vi "Configure AIN U6.vi"(4 "Binary":bool, 5 "Ranges":string[](array[string]), 6 "SettlingFactor":i32, 7 "Positive Channels":i32[](array[numeric]), 8 "error in":errorcluster, 10 "Resolution":i32, 11 "Handle In":i32) -> (0 "error out":errorcluster, 3 "Handle Out":i32)   [LabVIEW 2020]
panel:
  # "Pass an array of channels and range constants for\nthose channels."
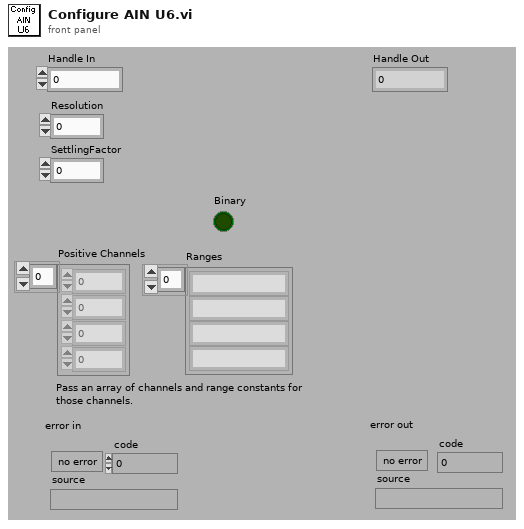
[diagram p1: front panel]
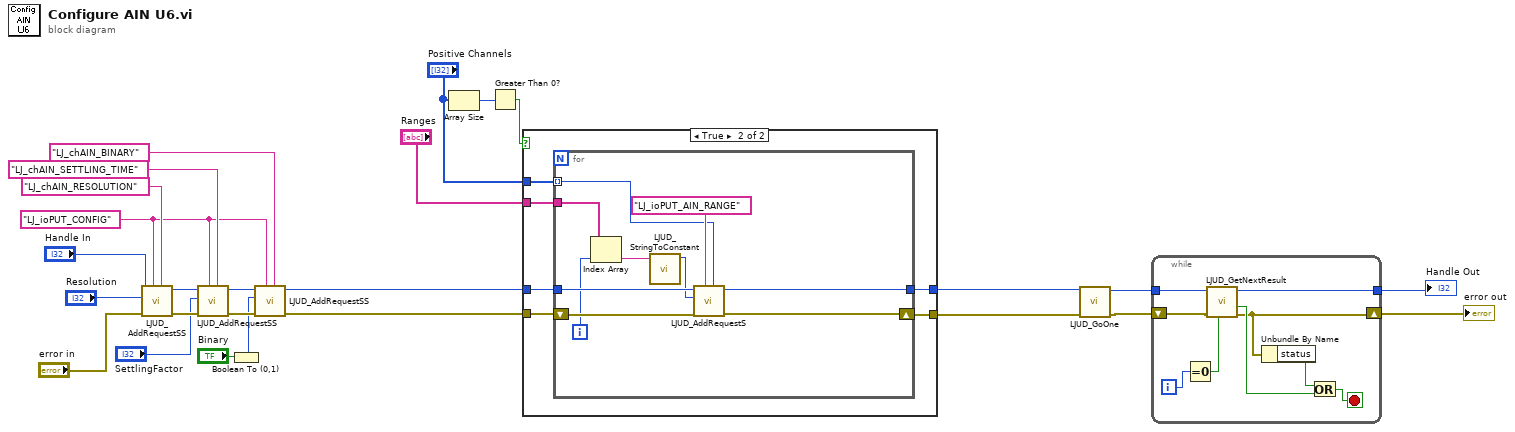
[diagram p0: block diagram]
diagram:
  w12 = "LJ_ioPUT_CONFIG" ("IOType")
  n1 = call "LJUD_AddRequestSS.vi"("Channel"="LJ_chAIN_RESOLUTION" ("IOType"), "IOType"=w12, "error in"="error in", "Value"="Resolution", "Handle In"="Handle In") -> ("error out"=w17:errorcluster, "Handle Out"=w19:i32)  [unwired: 5 in]
  n2 = call "LJUD_AddRequestSS.vi"("Channel"="LJ_chAIN_SETTLING_TIME" ("IOType"), "IOType"=w12, "error in"=w17, "Value"="SettlingFactor", "Handle In"=w19) -> ("error out"=w16:errorcluster, "Handle Out"=w18:i32)  [unwired: 5 in]
  n3 = Boolean To (0,1)(Boolean="Binary") -> (0, 1=w6:i16)
  n4 = call "LJUD_AddRequestSS.vi"("Channel"="LJ_chAIN_BINARY" ("IOType"), "IOType"=w12, "error in"=w16, "Value"=w6, "Handle In"=w18) -> ("error out"=w2:errorcluster, "Handle Out"=w3:i32)  [unwired: 5 in]
  n5 = Array Size(array="Positive Channels") -> (size(s)=w1:i32)
  n6 = Greater Than 0?(x=w1) -> (x > 0?=w23:bool)
  n7 = case shown="True" w23 {
    tunnel: w3 -> [w28 w34]
    tunnel: w2 -> [w27 w33]
    tunnel: "Positive Channels" -> [_ w32]
    tunnel: [w28 w29] -> w26
    tunnel: [w27 w31] -> w25
    tunnel: "Ranges" -> [_ w30]
    frame False {
    }
    frame True {
      n8 = for {
        tunnel: w34 -> [w44]
        shift-right: [w35] -> w31
        shift-left: w33 -> [w42]
        tunnel: w32 -> [w37] mode=indexing
        tunnel: w30 -> [w40]
        tunnel: [w36] -> w29
        i -> [w39]
        n9 = Index Array(array=w40, index=w39) -> (element=w38:string)
        n10 = call "LJUD_StringToConstant.vi"("String"=w38) -> ("Constant Number"=w41:i32)  [unwired: 9 in, 1 out]
        n11 = call "LJUD_AddRequestS.vi"("Channel"=w37, "IOType"="LJ_ioPUT_AIN_RANGE", "error in"=w42, "Value"=w41, "Handle In"=w44) -> ("error out"=w35:errorcluster, "Handle Out"=w36:i32)  [unwired: 5 in]
      }
    }
  }
  n12 = call "LJUD_GoOne.vi"("error in"=w25, "Handle In"=w26) -> ("error out"=w5:errorcluster, "Handle Out"=w22:i32)  [unwired: 8 in]
  n13 = while {
    shift-left: w5 -> [w46]
    shift-right: [w45] -> w4
    tunnel: [w49] -> w24
    tunnel: w22 -> [w51]
    i -> [w48]
    stop <- w53 stop-if-true
    n14 = Equal To 0?(x=w48) -> (x = 0?=w52:bool)
    n15 = call "LJUD_GetNextResult.vi"("GetFirst"=w52, "error in"=w46, "Handle In"=w51) -> ("error out"=w45:errorcluster, "LJE_NO_MORE_DATA_AVAILABLE"=w47:bool, "Handle Out"=w49:i32)  [unwired: 3 in, 3 out]
    n16 = Unbundle By Name(w45) -> ("status"=w50:bool)
    n17 = Or(x=w50, y=w47) -> (x .or. y?=w53:bool)
  }
  "Handle Out" <- w24
  "error out" <- w4
